vi "CAN Write.vi"(8 "error in (no error)":errorcluster, 10 "MessageBuffer":T1, 11 "Channel":u16) -> (0 "error out":errorcluster, 1 "Channel out":u16, 2 "MessageBuffer out":T1, 3 "function return":u32)   [LabVIEW 2025, in "PCAN2023.lvlib"]
doc: "Transmits a CAN message\n\n\nTPCANStatus __stdcall CAN_Write(\n TPCANHandle Channel, \n TPCANMsg* MessageBuffer);"
uses:
  PCAN2023.lvlib
  x64/PCANBasic.dll
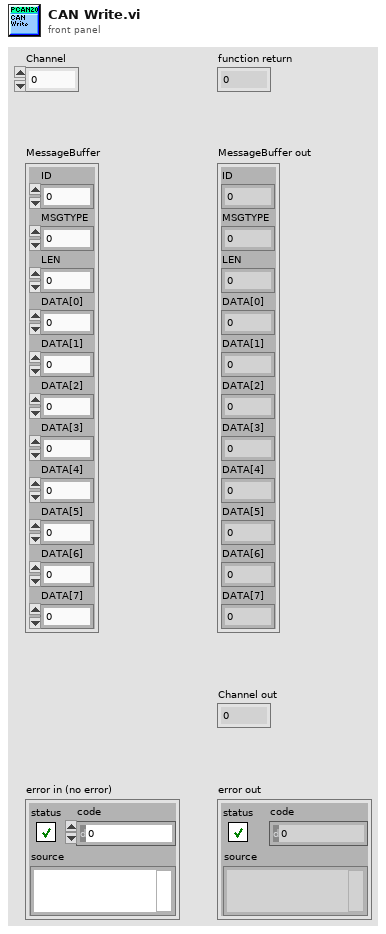
[diagram p1: front panel]
types:
  T1 = cluster{"ID":u32, "MSGTYPE":u8, "LEN":u8, "DATA[0]":u8, "DATA[1]":u8, "DATA[2]":u8, "DATA[3]":u8, "DATA[4]":u8, "DATA[5]":u8, "DATA[6]":u8, "DATA[7]":u8}
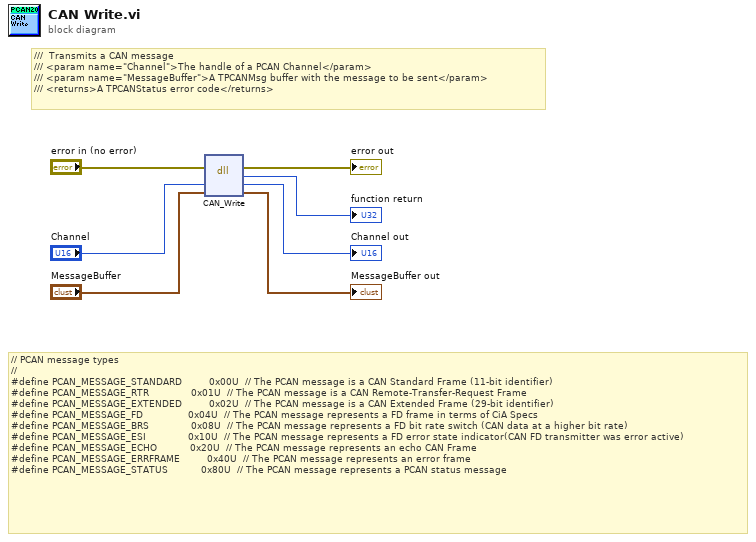
[diagram p0: block diagram]
diagram:
  # "// PCAN message types\n//\n#define PCAN_MESSAGE_STANDARD         0x00U  // The PCAN message is a CAN Standard Frame (11-bit identifier)\n#define PCAN_MESSAGE_RTR              0x01U  // The PCAN message is a CAN Remote-Transfer-Request Frame\n#define PCAN_MESSAGE_EXTENDED         0x02U  // The PCAN message is a CAN Extended Frame (29-bit identifier)\n#define PCAN_MESSAGE_FD               0x04U  // The PCAN message represents a FD frame in terms of CiA Specs\n#define PCAN_MESSAGE_BRS              0x08U  // The PCAN message represents a FD bit rate switch (CAN data at a higher bit rate)\n#define PCAN_MESSAGE_ESI              0x10U  // The PCAN message represents a FD error state indicator(CAN FD transmitter was error active)\n#define PCAN_MESSAGE_ECHO\t          0x20U  // The PCAN message represents an echo CAN Frame\n#define PCAN_MESSAGE_ERRFRAME         0x40U  // The PCAN message represents an error frame\n#define PCAN_MESSAGE_STATUS           0x80U  // The PCAN message represents a PCAN status message"
  # "///  Transmits a CAN message \n/// <param name=\"Channel\">The handle of a PCAN Channel</param>\n/// <param name=\"MessageBuffer\">A TPCANMsg buffer with the message to be sent</param>\n/// <returns>A TPCANStatus error code</returns>"
  n1 = dll-call lib="C:/UTP/LabView/Communication Handle/PCAN2023/x64/PCANBasic.dll" fn="CAN_Write"(error in="error in (no error)", "Channel"="Channel", "MessageBuffer"="MessageBuffer") -> (error out=→"error out":errorcluster, "return type"=→"function return":u32, "Channel"=→"Channel out":u16, "MessageBuffer"=→"MessageBuffer out":T1)  [unwired: 2 in, 1 out]
